vi "Maintain Caller Reference.vi"(7 "UID":i32, 11 "VI in":refnum<vi>) -> (3 "VI out":refnum<vi>)   [LabVIEW 2016, in "Assert API Components.lvlib"]
uses:
  Assert API Components.lvlib
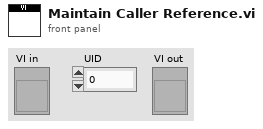
[diagram p1: front panel]
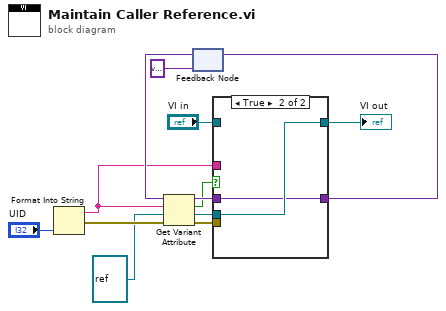
[diagram p0: block diagram]
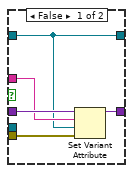
[diagram p2: hidden frame]
diagram:
  n1 = Format Into String("UID") -> (resulting string=w1:string, error out=w7:errorcluster)  [unwired: 3 in]
  n2 = feedback #1(variant) -> (w11:variant)
  n3 = Get Variant Attribute(Variant=w11, name=w1, default value (empty Variant)=refnum<vi> refnum ("Calling VI's Reference"), error in=w7) -> (duplicate Variant=w9:variant, found=w6:bool, value=w3:refnum<vi>, error out=w2:errorcluster)
  n4 = case shown="True" w6 {
    tunnel: [w17 w19] -> w12
    tunnel: w9 -> [w18 w19]
    tunnel: "VI in" -> [w14 _]
    tunnel: [w14 w20] -> w4
    tunnel: w3 -> [_ w20]
    tunnel: w2 -> [w15 _]
    tunnel: w1 -> [w16 _]
    frame False {
      n5 = Set Variant Attribute(Variant=w18, name=w16, value=w14, error in=w15) -> (Variant out=w17:variant)  [unwired: 2 out]
    }
    frame True {
    }
  }
  "VI out" <- w4
  n6 = feedback-in #1(w12) -> ()
